vi "dfd_Pos Imag.vi"(1 "complex in":cdb format="%.2f") -> (0 "complex out":cdb format="%.2f")   [LabVIEW 2017, in "NI_DigFilter_Design.lvlib"]
uses:
  <vilib>/addons/Digital Filter Design/NI_DigFilter_Design.lvlib
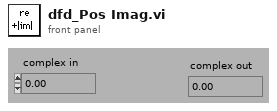
[diagram p1: front panel]
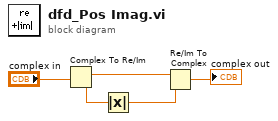
[diagram p0: block diagram]
diagram:
  n1 = Complex To Re/Im(x + iy="complex in") -> (x=w3:dbl, y=w4:dbl)
  n2 = Absolute Value(x=w4) -> (abs(x)=w2:dbl)
  n3 = Re/Im To Complex(1:w2, 2:w3) -> (0:→"complex out":cdb)
